vi "Execution_SetDebugOptions.vi"(8 "error in":errorcluster, 11 "EVE reference in":refnum<data-value>) -> (0 "error out":errorcluster, 3 "EVE reference out":refnum<data-value>)   [LabVIEW 2013, in "EVE.lvclass"]
uses:
  EVE.lvclass
  100_PROCESS/Class/Process/Process.lvclass
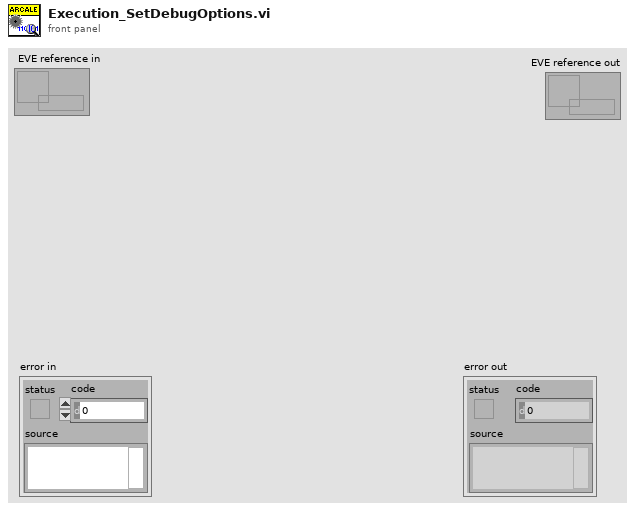
[diagram p1: front panel]
types:
  T1 = typedef "EVE.lvclass/CoreCluster.ctl" = cluster{"Events":cluster{"ToHmiSchedulerEvent":refnum<user-event>, "To Screens Event":refnum<user-event>, "ToAllProcessesEvent":refnum<user-event>, "ToProcessEvent":refnum<user-event>, "ToSplashScreenEvent":refnum<user-event>, "From Process Event":refnum<user-event>, "To message handler event":refnum<user-event>}, "Processes":T2}
  T2 = typedef "EVE.lvclass/Core_Processes-Cluster.ctl" = cluster{"List":refnum<class "Process.lvclass">[], "ProcessesRootPath":path}
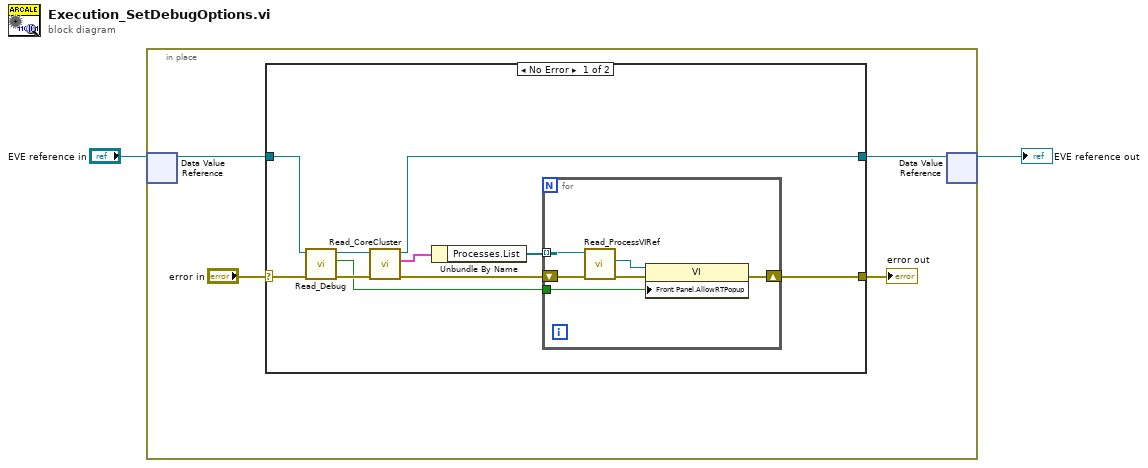
[diagram p0: block diagram]
diagram:
  n1 = in-place {
    n2 = in-place-dvr #1("EVE reference in") -> (w4:refnum<class "EVE.lvclass">)  [unwired: 1 out]
    n3 = case shown="No Error" "error in" {
      selector: "error in" -> [w16 w24]
      tunnel: [w9 w24] -> w5
      tunnel: [w12 w23] -> w3
      tunnel: w4 -> [w15 w23]
      frame No Error {
        n4 = call-dynamic "Read_Debug.vi"("error in (no error)"=w16, "EVE in"=w15) -> ("error out"=w14:errorcluster, "Debug ?"=w7:bool, "EVE out"=w13:refnum<class "EVE.lvclass">)  [unwired: 7 in]
        n5 = call-dynamic "Read_CoreCluster.vi"("Error In"=w14, "EVE in"=w13) -> ("Error out"=w8:errorcluster, "Core"=w11:T1, "EVE out"=w12:refnum<class "EVE.lvclass">)  [unwired: 7 in]
        n6 = Unbundle By Name(w11) -> ("Processes.List"=w10:refnum<class "Process.lvclass">[])
        n7 = for {
          tunnel: w10 -> [w21] mode=indexing
          shift-right: [w19] -> w9
          shift-left: w8 -> [w22]
          tunnel: w7 -> [w17]
          n8 = call-dynamic "Read_ProcessVIRef.vi"("error in (no error)"=w22, "Process in"=w21) -> ("error out"=w20:errorcluster, "Process VI Ref"=w18:refnum<vi>)  [unwired: 7 in, 1 out]
          n9 = property class="VI"(reference=w18, error in=w20, "Front Panel.AllowRTPopup"=w17) -> (error out=w19:errorcluster)  [unwired: 1 out]
        }
      }
      frame Error {
      }
    }
    "error out" <- w5
    n10 = in-place-dvr #1(w3) -> (→"EVE reference out":refnum<data-value>)  [unwired: 1 out]
  }
